vi "PPMS_Field_Step.vi"   [LabVIEW 2019]
uses:
  Global/Global Variables/global.vi
  Global/Global Variables/Data_Display_global.vi
  Instrument_Setup.vi
types:
  T1 = typedef "P9_P14_Magnet-cluster.ctl" = cluster{"Magnet (Oe)":dbl, "Setpoint (Oe)":dbl, "Rate (Oe/min)":dbl, "Set Field":bool, "Go to zero":bool, "Set Persitant/non-pers":bool, "Approach":i32, "Magnet Status":i32, "Sweeping":bool, "Quenched":bool, "Persitant Mode ":bool, "Stable":bool, "Steps":dbl, "Paused Menu":dbl, "B Step Start Field":dbl}
  T2 = typedef "P9P14_Magnet_Control.ctl" = cluster{"Setpoint (Oe)":dbl, "Rate (Oe/min)":dbl, "Set Field":bool, "Go to zero":bool, "Set Persitant/non-pers":bool, "Approach":i32, "Steps":dbl, "Paused Menu":dbl, "B Step start Field":dbl}
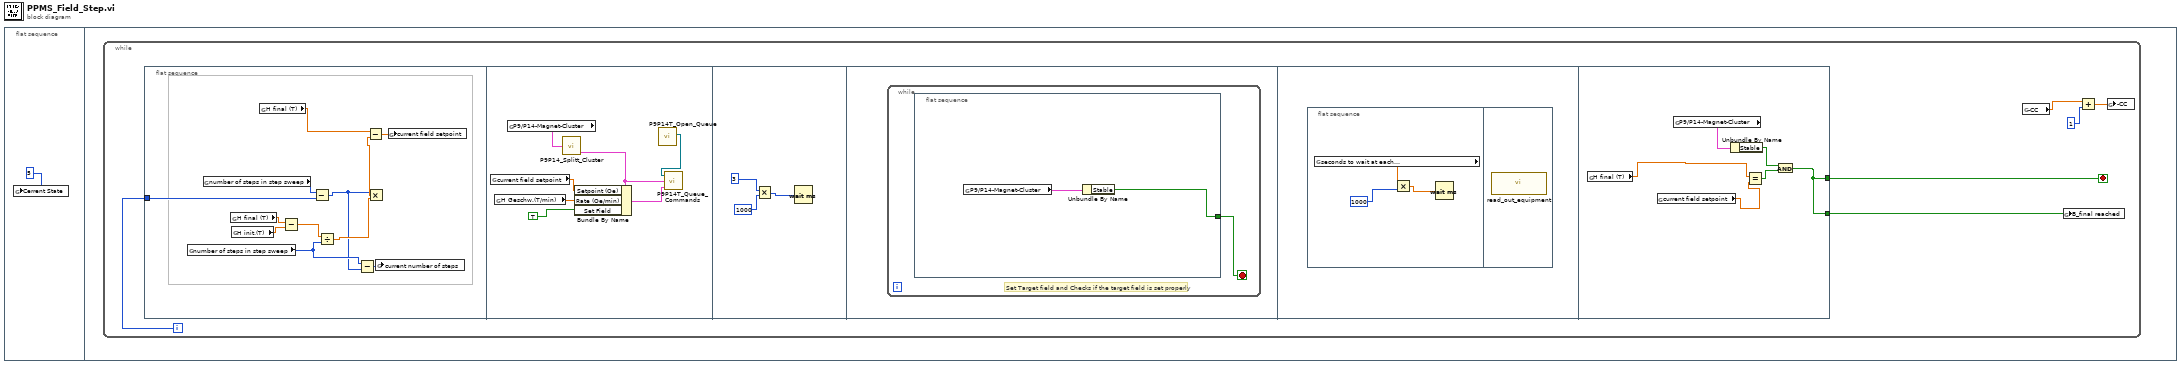
[diagram p0: block diagram]
diagram:
  n1 = flat-sequence {
    frame #0 {
      n2 = global write "global.vi" "Cerrent State"(5) -> ()
    }
    frame #1 {
      n3 = while {
        i -> [w7]
        stop <- w5 stop-if-true
        n4 = flat-sequence {
          tunnel: w7 -> [w8]
          tunnel: [w41] -> w6
          tunnel: [w41] -> w5
          frame #0 {
            n5 = global read "global.vi" "number of steps in step sweep"() -> (w13:i32)
            n6 = global read "global.vi" "number of steps in step sweep"() -> (w15:i32)
            n7 = global read "global.vi" "H final (T)"() -> (w11:dbl)
            n8 = global read "global.vi" "H init.(T)"() -> (w10:dbl)
            n9 = global read "global.vi" "H final (T)"() -> (w19:dbl)
            n10 = Subtract(x=w11, y=w10) -> (x-y=w9:dbl)
            n11 = Subtract(x=w15, y=w8) -> (x-y=w12:i32)
            n12 = Divide(x=w9, y=w13) -> (x/y=w17:dbl)
            n13 = Subtract(x=w13, y=w12) -> (x-y=w14:i32)
            n14 = Multiply(x=w12, y=w17) -> (x*y=w18:dbl)
            n15 = Subtract(x=w19, y=w18) -> (x-y=w16:dbl)
            n16 = global write "Data_Display_global.vi" "current number of steps"(w14) -> ()
            n17 = global write "Data_Display_global.vi" "current field setpoint"(w16) -> ()
          }
          frame #1 {
            n18 = global read "Data_Display_global.vi" "current field setpoint"() -> (w23:dbl)
            n19 = global read "global.vi" "H Geschw.(T/min)"() -> (w22:dbl)
            n20 = global read "Data_Display_global.vi" "P9/P14-Magnet-Cluster"() -> (w26:T1)
            n21 = call "P9P14_Splitt_Cluster.vi"("P9/P14-Magnet-Cluster"=w26) -> ("P9/P14-Magnet-Control"=w24:T2)  [unwired: 1 in, 1 out]
            n22 = Bundle By Name(cluster=w24, "Setpoint (Oe)"=w23, "Rate (Oe/min)"=w22, "Set Field"=TRUE) -> (w20:T2)
            n23 = call "P9P14T_Open_Queue.vi"() -> ("queue out"=w25:refnum<queue>)  [unwired: 10 in, 1 out]
            n24 = call "P9P14T_Queue_Commands.vi"("P9/P14-Magnet-Control"=w20, "P9/P14-Magnet-Control old status"=w24, "16T Queue"=w25) -> ()  [unwired: 1 out]
          }
          frame #2 {
            n25 = Multiply(x=3, y=1000) -> (x*y=w29:i32)
            n26 = Wait (ms)(milliseconds to wait=w29) -> ()  [unwired: 1 out]
          }
          frame #3 {
            n27 = while {
              stop <- w30 stop-if-true
              # "Set Target field and Checks if the target field is set properly"
              n28 = flat-sequence {
                tunnel: [w31] -> w30
                frame #0 {
                  n29 = global read "Data_Display_global.vi" "P9/P14-Magnet-Cluster"() -> (w32:T1)
                  n30 = Unbundle By Name(w32) -> ("Stable"=w31:bool)
                }
              }
            }
          }
          frame #4 {
            n31 = flat-sequence {
              frame #0 {
                n32 = global read "Instrument_Setup.vi" "seconds to wait at each\nfield step in a step sweep"() -> (w35:dbl)
                n33 = Multiply(x=w35, y=u32 1000 ("milliseconds to wait")) -> (x*y=w33:dbl)
                n34 = Wait (ms)(milliseconds to wait=w33) -> ()  [unwired: 1 out]
              }
              frame #1 {
                n35 = call "read_out_equipment.vi"() -> ()  [unwired: 1 in]
              }
            }
          }
          frame #5 {
            n36 = global read "global.vi" "H final (T)"() -> (w37:dbl)
            n37 = global read "Data_Display_global.vi" "current field setpoint"() -> (w36:dbl)
            n38 = global read "Data_Display_global.vi" "P9/P14-Magnet-Cluster"() -> (w40:T1)
            n39 = Unbundle By Name(w40) -> ("Stable"=w39:bool)
            n40 = Equal?(x=w37, y=w36) -> (x = y?=w38:bool)
            n41 = And(x=w39, y=w38) -> (x .and. y?=w41:bool)
          }
        }
        n42 = global read "global.vi" "-CC"() -> (w4:dbl)
        n43 = global write "Data_Display_global.vi" "B_final reached"(w6) -> ()
        n44 = Add(x=w4, y=1) -> (x+y=w2:dbl)
        n45 = global write "global.vi" "-CC"(w2) -> ()
      }
    }
  }
